vi "Insert_Into_Array.vi"(0 "Insert Into Array 1D":i8[](array[numeric])=[1, 2, 3, 4], 1 "Index IIA":i32, 2 "Element IIA":i8, 3 "SubArray IIA":i8[](array[numeric])=[-1, -2], 4 "Insert Into Array 2D":i8[][](array[numeric])=[[0, 3, 6], [1, 4, 7], [2, 5, 8]], 5 "Indexs IIA":T1={"Rows"=-1, "Columns"=-1}, 6 "SubArray IIA 2D":i8[][](array[numeric])=[[-10, -12], [-11, -13]], 8 "E or S IIA":T2, 10 "Choose IIA":T3) -> (21 "Array 1D IIA":i8[](array[numeric])=[1, 2, 3, 4], 25 "Array 2D IIA":i8[][](array[numeric]))   [LabVIEW 2018]
uses:
  Controls/1D_2D.ctl
  Controls/E_S.ctl
  Controls/Rows_Columns.ctl
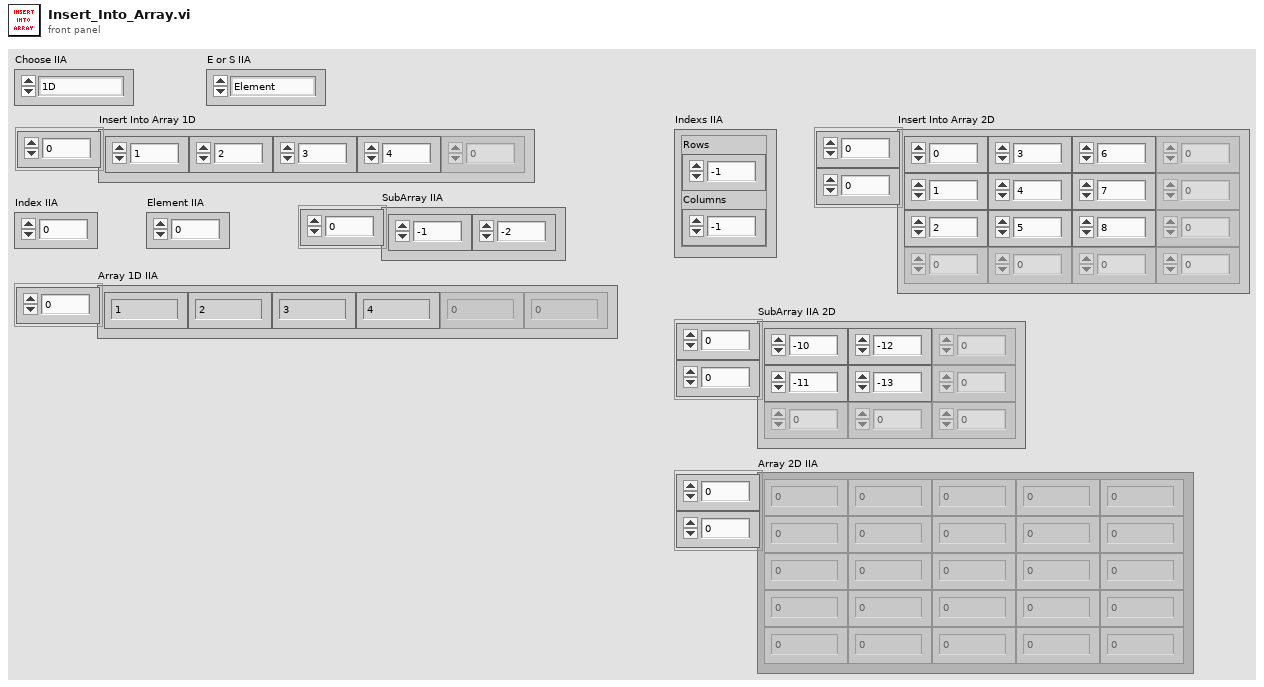
[diagram p1: front panel]
types:
  T1 = typedef "Rows_Columns.ctl" = cluster{"Rows":i32, "Columns":i32}
  T2 = typedef "E_S.ctl" = enum16{"Element", "SubArray"}
  T3 = typedef "1D_2D.ctl" = enum16{"1D", "2D"}
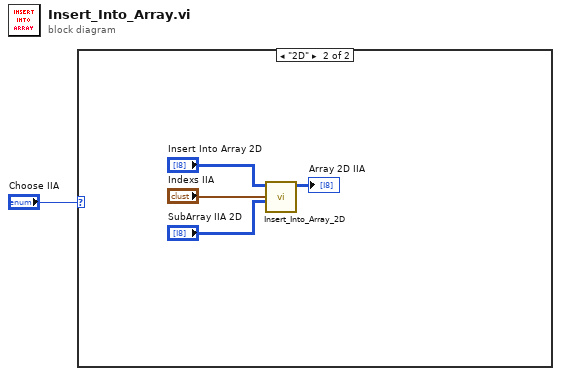
[diagram p0: block diagram]
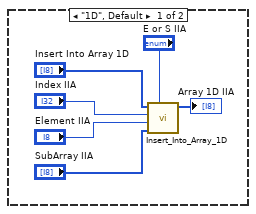
[diagram p2: hidden frame]
diagram:
  n1 = case shown="\"2D\"" "Choose IIA" {
    frame "1D", Default {
      n2 = call "Insert_Into_Array_1D.vi"("E or S IIA"="E or S IIA", "SubArray IIA"="SubArray IIA", "Element IIA"="Element IIA", "Index IIA"="Index IIA", "Insert Into Array 1D"="Insert Into Array 1D") -> ("Array 1D IIA"=→"Array 1D IIA":i8[])  [unwired: 6 in]
    }
    frame "2D" {
      n3 = call "Insert_Into_Array_2D.vi"("SubArray IIA 2D"="SubArray IIA 2D", "Indexs IIA"="Indexs IIA", "Insert Into Array 2D"="Insert Into Array 2D") -> ("Array 2D IIA"=→"Array 2D IIA":i8[][])  [unwired: 8 in]
    }
  }
